vi "line_follow.vi"(11 "New Heading":i16) -> (2 "output array":i16[](array[numeric]), 3 "x/y":i16)   [LabVIEW 2009]
panel:
  out "counter":i32
  out "x = y?":bool
  out "10 values":i16[](array[numeric])
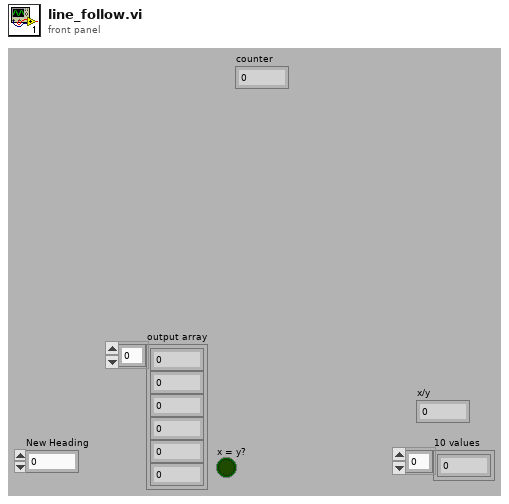
[diagram p1: front panel]
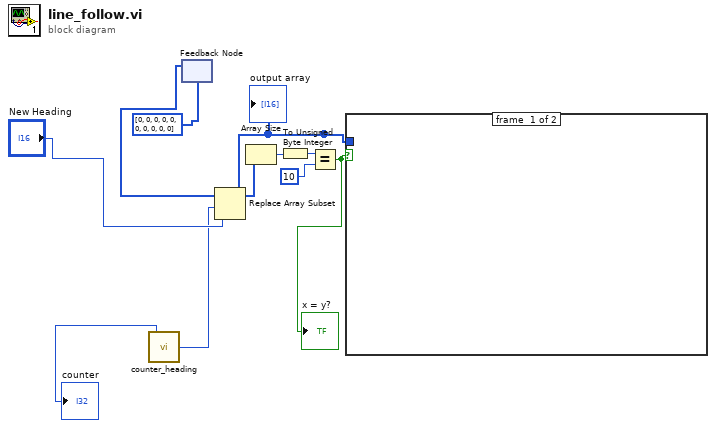
[diagram p0: block diagram]
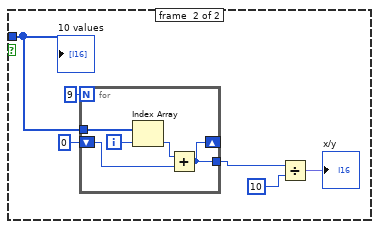
[diagram p2: hidden frame]
diagram:
  n1 = call "counter_heading.vi"() -> ("index"=w2:i32, "counter"=→"counter":i32)
  n2 = feedback #1(i16[] [0, 0, 0, 0, 0, 0, 0, 0, 0, 0]) -> (w3:i16[])
  n3 = Replace Array Subset(array=w3, new element="New Heading", index=w2) -> (w4:i16[])
  "output array" <- w4
  n4 = Array Size(array=w4) -> (size(s)=w7:i32)
  n5 = To Unsigned Byte Integer(number=w7) -> (unsigned 8bit integer=w6:u8)
  n6 = Equal?(x=w6, y=u8 10) -> (x = y?=w8:bool)
  "x = y?" <- w8
  n7 = case shown="True" w8 {
    tunnel: w4 -> [_ w12]
    frame #0 {
    }
    frame #1 {
      n8 = for {
        N: 9 -> [_]
        tunnel: w12 -> [w21]
        shift-right: [w17] -> _
        shift-left: i16 0 -> [w18]
        tunnel: [w17] -> w13
        i -> [w20]
        n9 = Index Array(array=w21, index=w20) -> (element=w19:i16)
        n10 = Add(x=w19, y=w18) -> (x+y=w17:i16)
      }
      n11 = Divide(x=w13, y=i16 10) -> (x/y=→"x/y":fxp<+/-,32,16>)
      "10 values" <- w12
    }
  }
